vi "Read Parity.vi"(8 "error in":errorcluster, 11 "ARINC 429 in":refnum<class "ARINC 429.lvclass">) -> (0 "error out":errorcluster, 2 "parity":enum16{"Even", "Odd"}(ring), 3 "ARINC 429 out":refnum<class "ARINC 429.lvclass">)   [LabVIEW 2020, in "ARINC 429.lvclass"]
uses:
  ARINC 429.lvclass
  ARINC 429.lvclass/ARINC 429.ctl
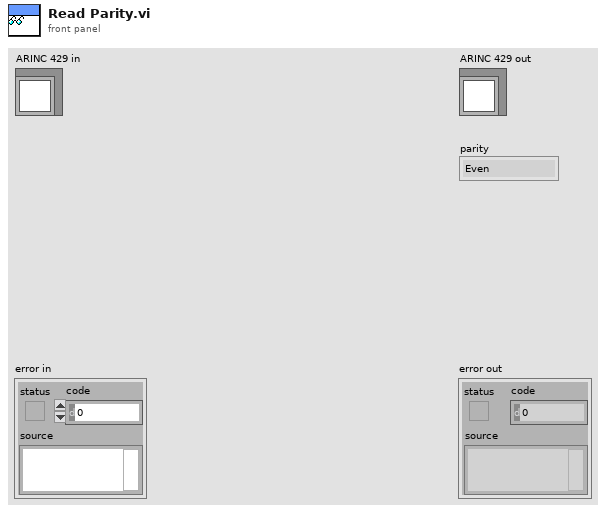
[diagram p1: front panel]
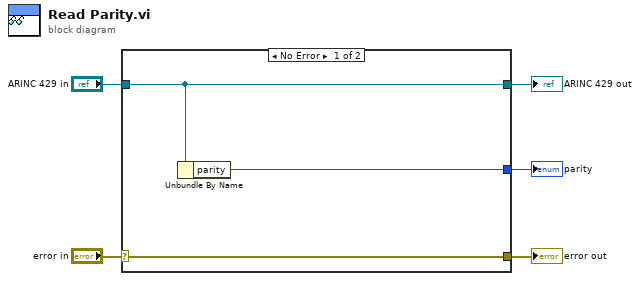
[diagram p0: block diagram]
diagram:
  n1 = case shown="No Error" "error in" {
    selector: "error in" -> [w8 w9]
    tunnel: [w8 w9] -> w4
    tunnel: [w7 w10] -> w2
    tunnel: "ARINC 429 in" -> [w7 w10]
    tunnel: [w6 _] -> w1
    frame No Error {
      n2 = Unbundle By Name(w7) -> ("parity"=w6:enum32{"Even", "Odd"})
    }
    frame Error {
    }
  }
  "error out" <- w4
  "ARINC 429 out" <- w2
  "parity" <- w1
